vi "ex14-8(subVI).vi"(1 "數值":dbl) -> (0 "溢位?":bool)   [LabVIEW 2014]
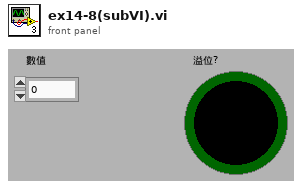
[diagram p1: front panel]
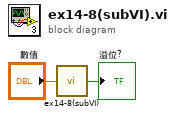
[diagram p0: block diagram]
diagram:
  n1 = call "ex14-8(subVI).vi"("數值"="數值") -> ("溢位?"=→"溢位?":bool)
